vi "GetVIText.vi"(8 "error in (no error)":errorcluster, 10 "Control Name (Blank = All controls in VI)":string, 11 "VI":refnum<vi>) -> (0 "error out":errorcluster, 1 "Font Name":string, 2 "Control Text":string[](array[string]), 3 "Control Keys":string[](array[string]), 5 "number_of_records":i32)   [LabVIEW 2019]
uses:
  <vilib>/Utility/traverseref.llb/TRef TravTarget.ctl
  <vilib>/Utility/traverseref.llb/VI Scripting - Traverse.lvlib
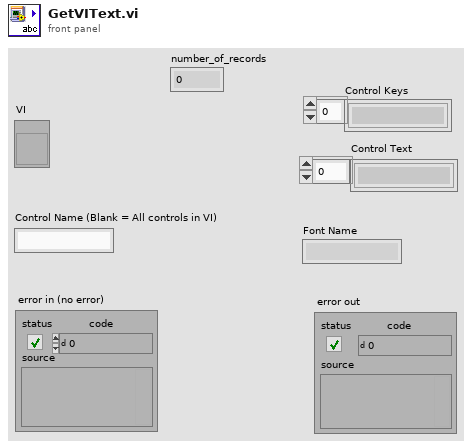
[diagram p1: front panel]
types:
  T1 = typedef "TRef TravTarget.ctl" = enum16{"FP", "BD", "Other"}
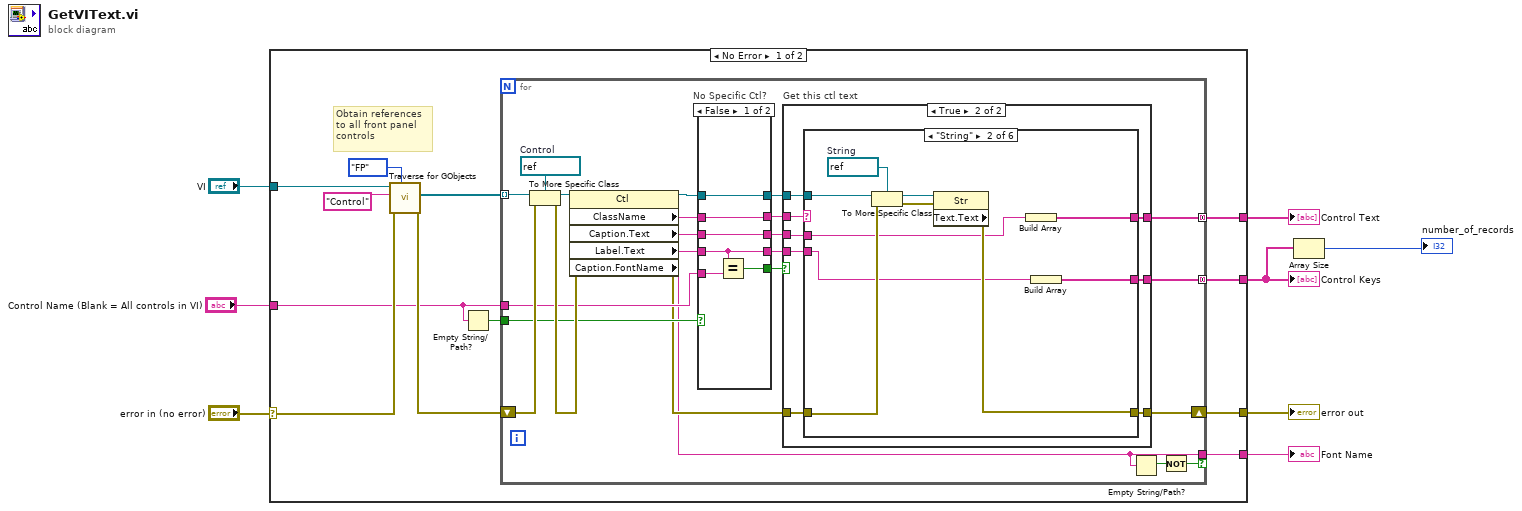
[diagram p0: block diagram]
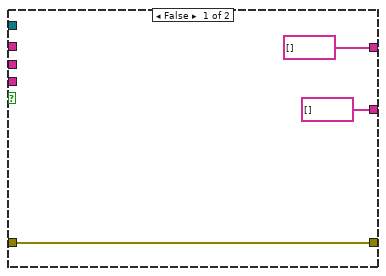
[diagram p2: hidden frame]
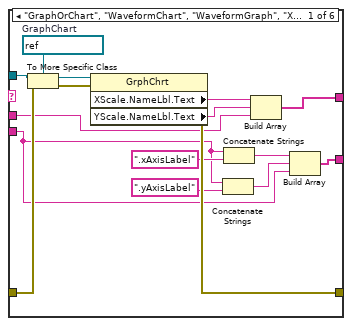
[diagram p3: hidden frame]
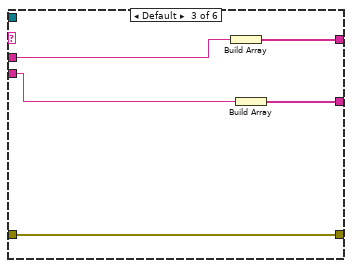
[diagram p4: hidden frame]
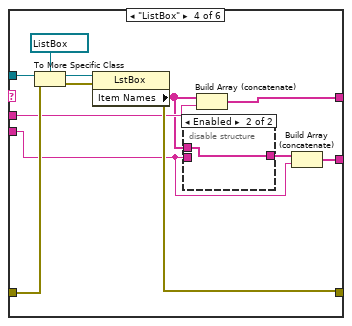
[diagram p5: hidden frame]
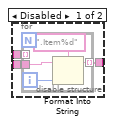
[diagram p6: hidden frame]
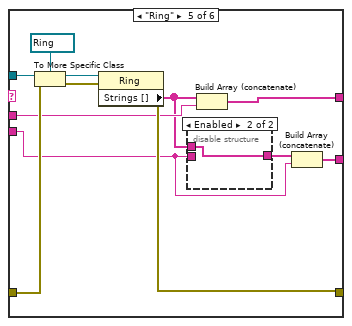
[diagram p7: hidden frame]
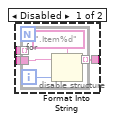
[diagram p8: hidden frame]
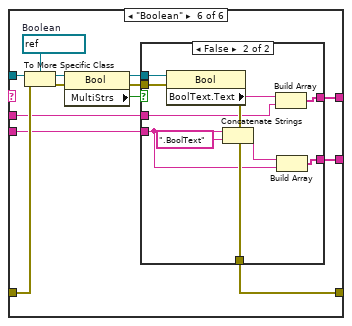
[diagram p9: hidden frame]
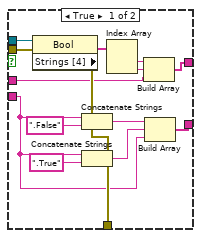
[diagram p10: hidden frame]
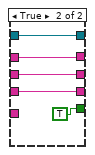
[diagram p11: hidden frame]
diagram:
  n1 = case shown="No Error" "error in (no error)" {
    selector: "error in (no error)" -> [w16 w174]
    tunnel: "VI" -> [w18 _]
    tunnel: "Control Name (Blank = All controls in VI)" -> [w12 _]
    tunnel: [w14 w174] -> w5
    tunnel: [w11 _] -> w4
    tunnel: [w10 _] -> w2
    tunnel: [w9 _] -> w3
    frame No Error {
      # "Obtain references to all front panel controls"
      n2 = call <vilib>:"Traverse for GObjects.vi"("Traverse Target"=TRef_TravTarget."FP", "error in (no error)"=w16, "Class Name"="Control", "VI Refnum"=w18) -> ("error out"=w15:errorcluster, "References"=w17:refnum<vi>[])  [unwired: 4 in, 2 out]
      n3 = Empty String/Path?(string/path=w12) -> (empty?=w13:bool)
      n4 = for {
        tunnel: w17 -> [w43] mode=indexing
        shift-right: [w32] -> w14
        shift-left: w15 -> [w40]
        tunnel: w12 -> [w38]
        tunnel: w13 -> [w36]
        tunnel: [w25] -> w11 mode=concatenating
        tunnel: [w24] -> w10 mode=concatenating
        tunnel: [w23] -> w9 if=w21
        w41 = refnum<vi> refnum  # Control
        n5 = To More Specific Class(target class=w41, reference=w43, error in=w40) -> (specific class reference=w42:refnum<vi>, error out=w39:errorcluster)
        n6 = property class="Ctl"(reference=w42, error in=w39) -> (reference out=w26:refnum<vi>, error out=w33:errorcluster, "ClassName"=w35:string, "Caption.Text"=w34:string, "Label.Text"=w37:string, "Caption.FontName"=w23:string)
        n7 = case "No Specific Ctl?" shown="False" w36 {
          tunnel: w38 -> [w168 _]
          tunnel: w37 -> [w166 w170]
          tunnel: w35 -> [w164 w173]
          tunnel: w34 -> [w165 w171]
          tunnel: [w167 TRUE] -> w31
          tunnel: [w164 w173] -> w28
          tunnel: [w165 w171] -> w30
          tunnel: [w166 w170] -> w29
          tunnel: [w163 w169] -> w27
          tunnel: w26 -> [w163 w169]
          frame False {
            n8 = Equal?(x=w166, y=w168) -> (x = y?=w167:bool)
          }
          frame True {
          }
        }
        n9 = case "Get this ctl text" shown="True" w31 {
          tunnel: w33 -> [w46 w52]
          tunnel: [w46 w51] -> w32
          tunnel: w30 -> [_ w49]
          tunnel: w29 -> [_ w50]
          tunnel: w28 -> [_ w54]
          tunnel: w27 -> [_ w53]
          tunnel: [string[] [] w48] -> w25
          tunnel: [string[] [] w47] -> w24
          frame False {
          }
          frame True {
            n10 = case shown="\"String\"" w54 {
              tunnel: w53 -> [w67 w77 _ w94 w114 w137]
              tunnel: w52 -> [w66 w76 w85 w93 w113 w136]
              tunnel: [w65 w75 w85 w92 w112 w135] -> w51
              tunnel: [w64 w74 w84 w91 w111 w134] -> w48
              tunnel: w50 -> [w56 w72 w82 w87 w107 w132]
              tunnel: w49 -> [w63 w73 w83 w90 w110 w133]
              tunnel: [w55 w71 w81 w86 w106 w131] -> w47
              frame "GraphOrChart", "WaveformChart", "WaveformGraph", "XYGraph" {
                w69 = refnum<vi> refnum  # GraphChart
                n11 = To More Specific Class(target class=w69, reference=w67, error in=w66) -> (specific class reference=w70:refnum<vi>, error out=w68:errorcluster)
                n12 = property class="GrphChrt"(reference=w70, error in=w68) -> (error out=w65:errorcluster, "XScale.NameLbl.Text"=w60:string, "YScale.NameLbl.Text"=w59:string)  [unwired: 1 out]
                n13 = Concatenate Strings(w56, ".yAxisLabel" ("string")) -> (w57:string)
                n14 = Concatenate Strings(w56, ".xAxisLabel" ("string")) -> (w58:string)
                n15 = Build Array(w60, w59, w63) -> (w64:string[])
                n16 = Build Array(w58, w57, w56) -> (w55:string[])
              }
              frame "String" {
                w80 = refnum<vi> refnum  # String
                n17 = To More Specific Class(target class=w80, reference=w77, error in=w76) -> (specific class reference=w79:refnum<vi>, error out=w78:errorcluster)
                n18 = property class="Str" props=["Text", "Text"](reference=w79, error in=w78) -> (error out=w75:errorcluster)  [unwired: 2 out]
                n19 = Build Array(w73) -> (w74:string[])
                n20 = Build Array(w72) -> (w71:string[])
              }
              frame Default {
                n21 = Build Array(w83) -> (w84:string[])
                n22 = Build Array(w82) -> (w81:string[])
              }
              frame "ListBox" {
                n23 = To More Specific Class(target class=refnum<vi> refnum ("reference out"), reference=w94, error in=w93) -> (specific class reference=w97:refnum<vi>, error out=w96:errorcluster)
                n24 = property class="LstBox"(reference=w97, error in=w96) -> (error out=w92:errorcluster, "Item Names"=w89:string[])  [unwired: 1 out]
                n25 = disable-structure shown="Enabled" {
                  disable-tunnel: w89 -> [w100 w105]
                  disable-tunnel: [w99 w105] -> w88
                  disable-tunnel: w87 -> [w98 _]
                  frame Disabled {
                    n26 = for {
                      tunnel: w98 -> [w104]
                      tunnel: w100 -> [_] mode=indexing
                      tunnel: [w101] -> w99 mode=indexing
                      i -> [w102]
                      n27 = Format Into String(format string=".Item%d", initial string=w104, w102) -> (resulting string=w101:string)  [unwired: 1 in, 1 out]
                    }
                  }
                  frame Enabled {
                  }
                }
                n28 = Build Array (concatenate)(w89, w90) -> (w91:string[])
                n29 = Build Array (concatenate)(w88, w87) -> (w86:string[])
              }
              frame "Ring" {
                n30 = To More Specific Class(target class=refnum<vi> refnum ("reference out"), reference=w114, error in=w113) -> (specific class reference=w117:refnum<vi>, error out=w116:errorcluster)
                n31 = property class="Ring"(reference=w117, error in=w116) -> (error out=w112:errorcluster, "Strings []"=w109:string[])  [unwired: 1 out]
                n32 = disable-structure shown="Enabled" {
                  disable-tunnel: w109 -> [w120 w125]
                  disable-tunnel: [w119 w125] -> w108
                  disable-tunnel: w107 -> [w118 _]
                  frame Disabled {
                    n33 = for {
                      tunnel: w118 -> [w124]
                      tunnel: w120 -> [_] mode=indexing
                      tunnel: [w121] -> w119 mode=indexing
                      i -> [w122]
                      n34 = Format Into String(format string=".Item%d", initial string=w124, w122) -> (resulting string=w121:string)  [unwired: 1 in, 1 out]
                    }
                  }
                  frame Enabled {
                  }
                }
                n35 = Build Array (concatenate)(w109, w110) -> (w111:string[])
                n36 = Build Array (concatenate)(w108, w107) -> (w106:string[])
              }
              frame "Boolean" {
                w138 = refnum<vi> refnum  # Boolean
                n37 = To More Specific Class(target class=w138, reference=w137, error in=w136) -> (specific class reference=w130:refnum<vi>, error out=w128:errorcluster)
                n38 = property class="Bool"(reference=w130, error in=w128) -> (reference out=w129:refnum<vi>, error out=w127:errorcluster, "MultiStrs"=w126:bool)
                n39 = case shown="False" w126 {
                  tunnel: [w152 w157] -> w135
                  tunnel: [w150 w161] -> w134
                  tunnel: w133 -> [w139 w153]
                  tunnel: w132 -> [w145 w154]
                  tunnel: [w144 w160] -> w131
                  tunnel: w129 -> [w143 w159]
                  tunnel: w127 -> [w142 w158]
                  frame True {
                    n40 = property class="Bool"(reference=w143, error in=w142) -> (error out=w152:errorcluster, "Strings [4]"=w151:string[])  [unwired: 1 out]
                    n41 = Concatenate Strings(w145, ".False" ("string")) -> (w148:string)
                    n42 = Concatenate Strings(w145, ".True" ("string")) -> (w146:string)
                    n43 = Index Array(array=w151) -> (element #1=w141:string, element #2=w140:string)  [unwired: 2 in]
                    n44 = Build Array(w141, w140, w139) -> (w150:string[])
                    n45 = Build Array(w148, w146, w145) -> (w144:string[])
                  }
                  frame False {
                    n46 = property class="Bool"(reference=w159, error in=w158) -> (error out=w157:errorcluster, "BoolText.Text"=w162:string)  [unwired: 1 out]
                    n47 = Concatenate Strings(w154, ".BoolText" ("string")) -> (w156:string)
                    n48 = Build Array(w162, w153) -> (w161:string[])
                    n49 = Build Array(w156, w154) -> (w160:string[])
                  }
                }
              }
            }
          }
        }
        n50 = Empty String/Path?(string/path=w23) -> (empty?=w22:bool)
        n51 = Not(x=w22) -> (.not. x?=w21:bool)
      }
    }
    frame Error {
    }
  }
  "Control Text" <- w4
  "error out" <- w5
  "Control Keys" <- w2
  "Font Name" <- w3
  n52 = Array Size(array=w2) -> (size(s)=→"number_of_records":i32)
